vi "1B_BufferPulseTrain.vi"(0 "Waveform In":waveform(dbl)={"t0"=timestamp(3462203691.797 s since 1904-01-01), "dt"=1.428e-05, "Y"=array[8000 elements]}, 2 "Mode":enum16{"init", "Add", "Read"}(ring), 11 "error in":errorcluster) -> (4 "Array":waveform(dbl)[](array[waveform]), 15 "error out":errorcluster)   [LabVIEW 2010]
panel:
  in  "Show Graph":bool
  out "XY Graph":cluster{dbl[], dbl[]}[](graph)
  # "Tip: Select \"Simple\" if \"Precise\" cannot mesure offset"
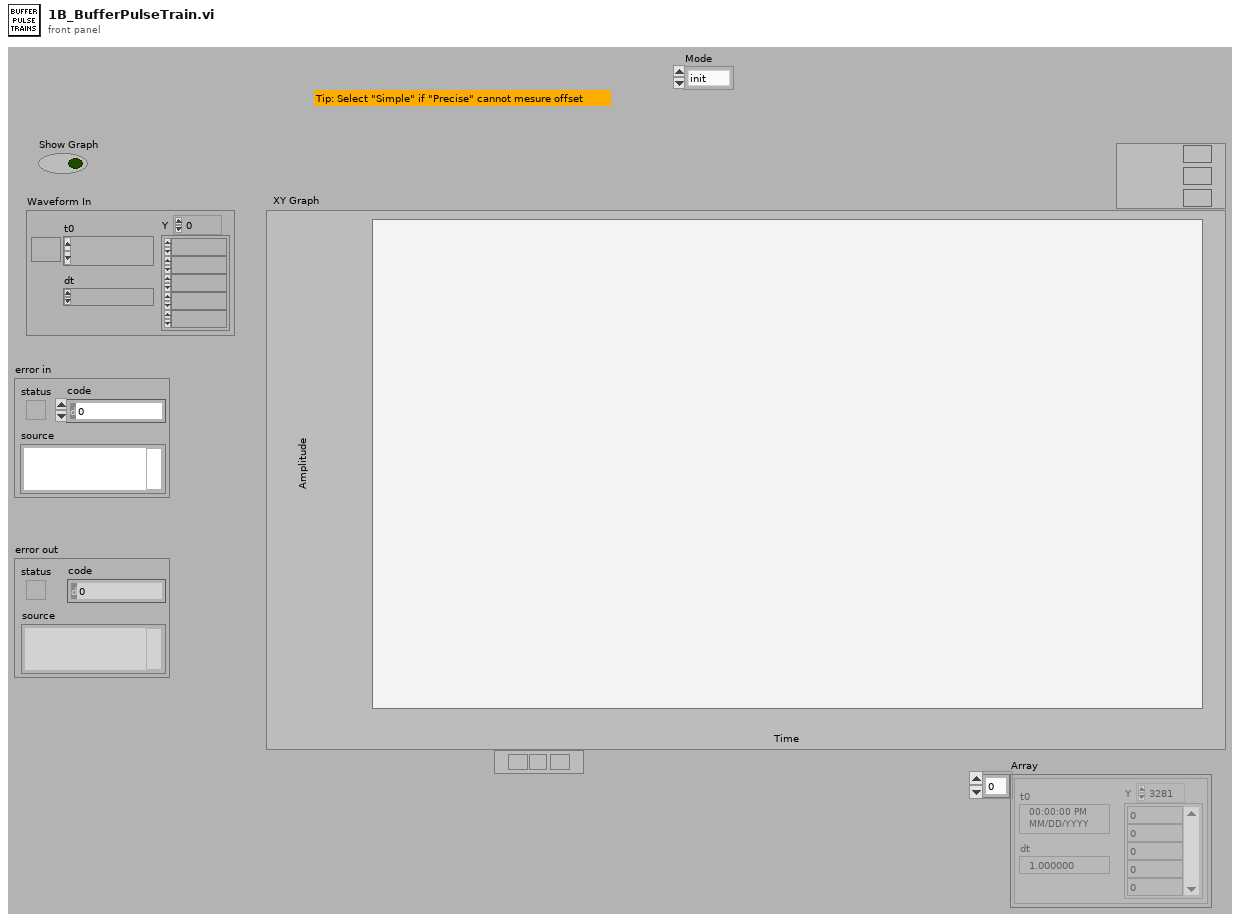
[diagram p1: front panel]
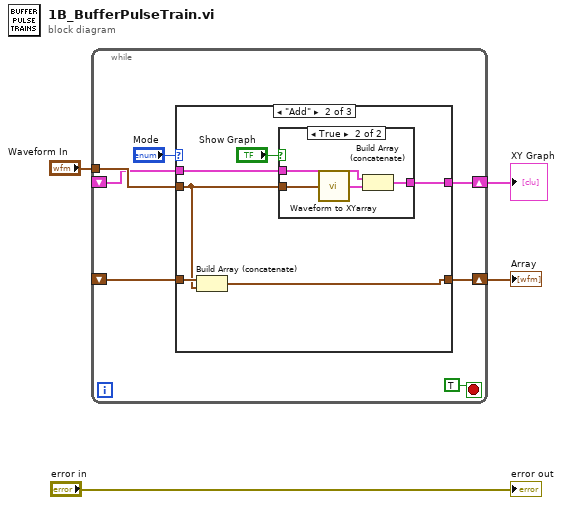
[diagram p0: block diagram]
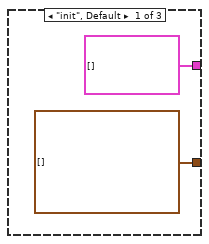
[diagram p2: hidden frame]
diagram:
  n1 = while {
    shift-right: [w8] -> w3
    shift-left: _ -> [w9]
    tunnel: "Waveform In" -> [w10]
    shift-right: [w5] -> w2
    shift-left: _ -> [w6]
    stop <- TRUE stop-if-true
    n2 = case shown="\"Add\"" "Mode" {
      tunnel: [cluster{"X array":dbl[], "Y array":dbl[]}[] [] ("appended array") w19 w26] -> w8
      tunnel: w10 -> [_ w15 _]
      tunnel: w9 -> [_ w18 w26]
      tunnel: w6 -> [_ w17 w25]
      tunnel: [waveform(dbl)[] [] w16 w25] -> w5
      frame "init", Default {
      }
      frame "Add" {
        n3 = Build Array (concatenate)(w17, w15) -> (w16:waveform(dbl)[])
        n4 = case shown="True" "Show Graph" {
          tunnel: [w20 w24] -> w19
          tunnel: w18 -> [w20 w23]
          tunnel: w15 -> [_ w21]
          frame False {
          }
          frame True {
            n5 = call "Waveform to XYarray.vi"("Waveform In"=w21) -> ("Single Plot"=w22:cluster{"X array":dbl[], "Y array":dbl[]})
            n6 = Build Array (concatenate)(w23, w22) -> (w24:cluster{"X array":dbl[], "Y array":dbl[]}[])
          }
        }
      }
      frame "Read" {
      }
    }
  }
  "XY Graph" <- w3
  "Array" <- w2
  "error out" <- "error in"
